vi "Q&E Base string.vi"(0 "E&S Message":T1) -> ()   [LabVIEW 2011]
uses:
  Application Structure/E&S Note ID.ctl
  emi Lib/System 01/0 - General/S&E reporting/Private/_emi_ S&E Message note.ctl
  <vilib>/Utility/VariantDataType/VariantType.lvlib
  <vilib>/Utility/VariantDataType/Type.ctl
  emi Lib/System 01/0 - General/S&E reporting/Private/_emi_ S&E Message type.ctl
  emi Lib/System 01/0 - General/S&E reporting/Private/_emi_ S&E Message.ctl
panel:
  out "format string":string
  in  "Note":variant
  in  "Delimiter(;)":string=";"
  out "resulting string":string
  in  "Delimiter_(;)":string=";"
  in  "Time format(%T)":string="%T"
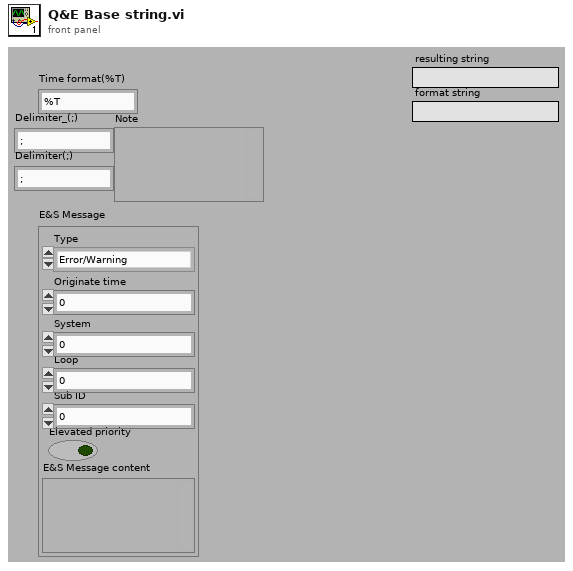
[diagram p1: front panel]
types:
  T1 = typedef "_emi_ S&E Message.ctl" = cluster{"Type":T2, "Originate time":dbl, "System":u8, "Loop":u16, "Sub ID":u16, "Elevated priority":bool, "E&S Message content":variant}
  T2 = typedef "_emi_ S&E Message type.ctl" = enum16{"Error/Warning", "Note", "Debug", "Event", "Alarm Analog", "Alarm Digital", "Annotation"}
  T3 = typedef "VariantType.lvlib/Type.ctl" = enum8{"Invalid Type", "Void", "I8", "I16", "I32", "I64", "U8", "U16", "U32", "U64", "Single Float", "Double Float", "Extended Float", "Single Complex", "Double Complex", "Extended Complex", "Enum U8", "Enum U16", "Enum U32", "Enum U64", "Single Float With Unit", "Double Float With Unit", "Extended Float With Unit", "Single Complex with Unit", "Double Complex with Unit", "Extended Complex with Unit", "Boolean", "String", "Path", "Picture", "Tag", "Array", "Cluster", "Variant", "LV Variant", "Waveform", "Timestamp", "Digital Waveform", "Digital Data", "ExpressData", "Refnum", "External Data", "VI", "Poly VI", "LabVIEW Class Instance", "Fixed Point"}
  T4 = typedef "_emi_ S&E Message note.ctl" = cluster{"Note ID":i16, "Note":string}
  T5 = typedef "E&S Note ID.ctl" = enum16{"Program Started", "Program terminated", "User Changed", "General information"}
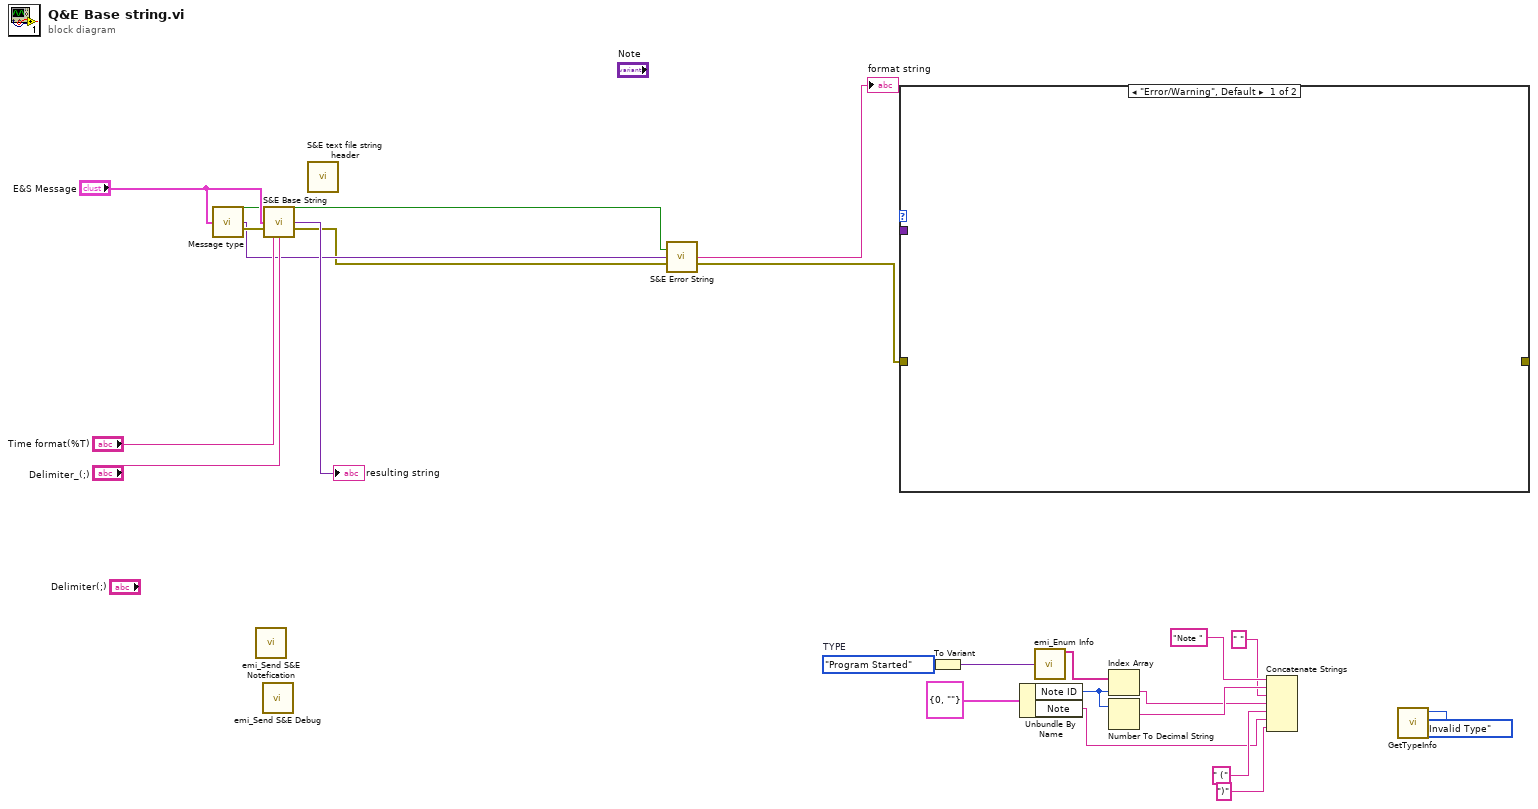
[diagram p0: block diagram]
diagram:
  w21 = E&S_Note_ID."Program Started"  # TYPE
  n1 = call "Message type.vi"("E&S Message"="E&S Message") -> ("Elevated priority"=w3:bool, "Content"=w6:variant, "error out"=w8:errorcluster)  [unwired: 11 in, 1 out]
  n2 = call "emi_Send S&E Notefication.vi"() -> ()  [unwired: 14 in, 2 out]
  n3 = call "emi_Send S&E Debug.vi"() -> ()  [unwired: 14 in, 2 out]
  n4 = call "S&E Base String.vi"("E&S Message"="E&S Message", "error in (no error)"=w8, "Time format(%T)"="Time format(%T)", "Sub ID"="Delimiter_(;)") -> ("Message content"=→"resulting string":variant, "error out"=w5:errorcluster)  [unwired: 5 in, 5 out]
  n5 = call "S&E text file string header.vi"() -> ()  [unwired: 13 in, 3 out]
  n6 = call "S&E Error String.vi"("Elevated priority"=w3, "Content"=w6, "error in"=w5) -> ("format string"=→"format string":string, "error out"=w4:errorcluster)  [unwired: 11 in]
  n7 = case shown="\"Error/Warning\", Default" {
    selector: _ -> [_ _]
    tunnel: w4 -> [w26 _]
    tunnel: _ -> [w25 _]
    tunnel: _ -> [w24 _]
    frame "Error/Warning", Default {
    }
    frame "Note" {
    }
  }
  n8 = To Variant(anything=w21) -> (Variant=w20:variant)
  n9 = Unbundle By Name(T4 {"Note ID"=0, "Note"=""} ("E&S Note")) -> ("Note ID"=w17:i16, "Note"=w10:string)
  n10 = call "emi_Enum Info.vi"("Enum"=w20) -> ("Text Elements"=w19:string[])  [unwired: 11 in, 3 out]
  n11 = Index Array(array=w19, index=w17) -> (element=w13:string)
  n12 = Number To Decimal String(number=w17) -> (decimal integer string=w15:string)  [unwired: 1 in]
  n13 = Concatenate Strings("Note " ("string"), w15, " " ("string"), w13, " (" ("string"), w10, ")" ("string")) -> ()  [unwired: 1 out]
  n14 = call <vilib>:"GetTypeInfo.vi"() -> ("Type Enum"=w1:T3)  [unwired: 7 in, 4 out]
